vi "Save and Load Fixed-Point Settings.vi"() -> ()   [LabVIEW 2019]
doc: "This example demonstrates how to simulate the performance of a fixed-point LMS adaptive filter, obtain appropriate fixed-point settings from the simulation, save these settings to an XML file, and then load that XML file into LabVIEW.\n\nComplete the following steps to use this example.\n\n1. Select <b>Save to File</b> from the <b>Operation</b> pull-down menu and run this VI.\n\n2. In the dialog box that appears, specify a file name and click the <b>OK</b> button to save the fixed-point settings.\n\n3. Close and reopen this example.\n\n4. Select <b>Load from File</b> from the <b>Operation</b> pull-down menu and run this VI.\n \n5. In the dialog box that appears, navigate to the XML file you saved in Step 2 and click the <b>Open</b> button. This example then loads the fixed-point settings and displays the settings in <b>Fixed-Point Settings</b>."
uses:
  <vilib>/addons/Adaptive Filters/Utilities/AFT Fixed-Point Settings.ctl
  <vilib>/addons/Adaptive Filters/Utilities/AFT Algorithm.ctl
  <vilib>/addons/Adaptive Filters/Fixed-Point Simulation/LMS/AFT Simulate Fixed-Point FIR LMS.xnode
  <vilib>/addons/Adaptive Filters/NI_AdaptiveFilter.lvlib
  <vilib>/addons/Adaptive Filters/Utilities/AFT Simulation Info.ctl
panel:
  in  "Operation":enum16{"Save to File", "Load from File"}(ring)
  out "Coefficients":dbl[][](graph)
  out "Fixed-Point Settings":T1 {"algorithm" items=["LMS"]}
  out "Error Signal":dbl[](graph)
  # "Select Help>>Show Context Help and move the cursor over the VI icon of this example for more information."
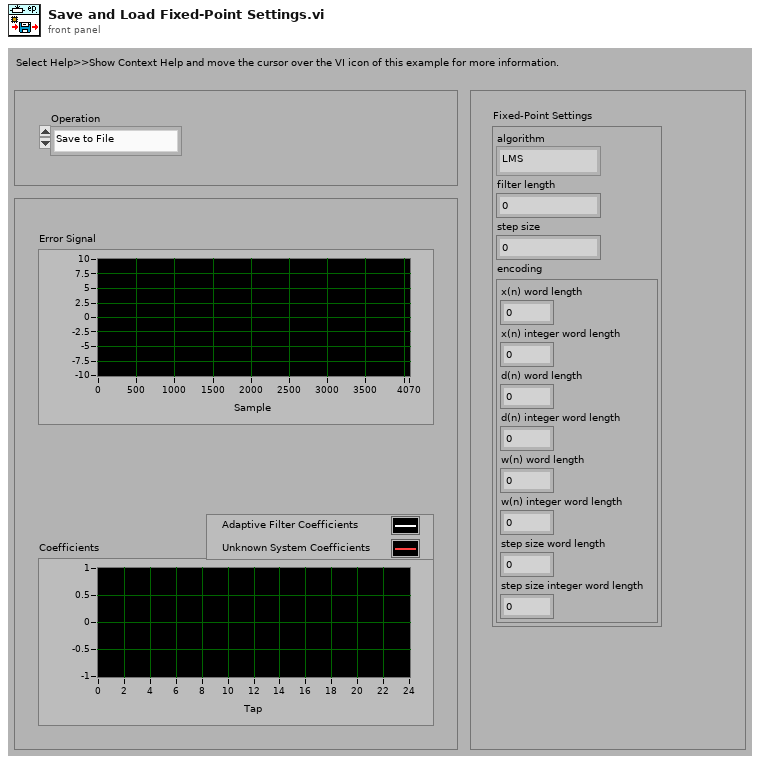
[diagram p1: front panel]
types:
  T1 = cluster{"algorithm":u16, "filter length":i32, "step size":dbl, "encoding":cluster{"x(n) word length":i32, "x(n) integer word length":i32, "d(n) word length":i32, "d(n) integer word length":i32, "w(n) word length":i32, "w(n) integer word length":i32, "step size word length":i32, "step size integer word length":i32}}
  T2 = typedef "NI_AdaptiveFilter.lvlib/AFT Fixed-Point Settings.ctl" = cluster{"algorithm":u16, "filter length":i32, "step size":dbl, "encoding":cluster{"x(n) word length":i32, "x(n) integer word length":i32, "d(n) word length":i32, "d(n) integer word length":i32, "w(n) word length":i32, "w(n) integer word length":i32, "step size word length":i32, "step size integer word length":i32}}
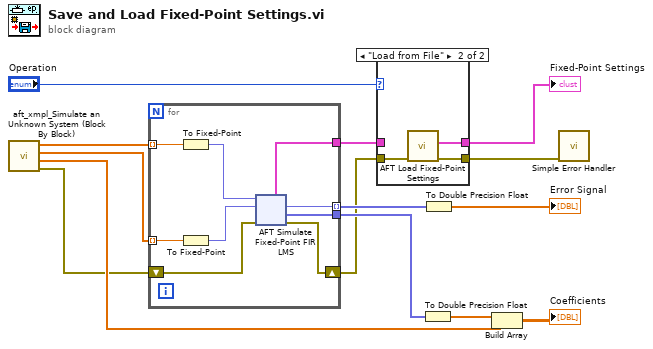
[diagram p0: block diagram]
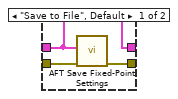
[diagram p2: hidden frame]
diagram:
  n1 = call "aft_xmpl_Simulate an Unknown System (Block By Block).vi"() -> ("error out"=w4:errorcluster, "unknown system coefficients"=w5:dbl[], "response signal"=w6:dbl[], "stimulus signal"=w7:dbl[])  [unwired: 4 in, 4 out]
  n2 = for {
    tunnel: w7 -> [w20] mode=indexing
    tunnel: w6 -> [w21] mode=indexing
    tunnel: [w23] -> w14 mode=indexing
    tunnel: [w22] -> w12
    tunnel: [w17] -> w11
    shift-right: [w16] -> w8
    shift-left: w4 -> [w15]
    n3 = To Fixed-Point(number=w20) -> (fixed-point=w19:fxp<+/-,24,4>)  [unwired: 1 out]
    n4 = To Fixed-Point(number=w21) -> (fixed-point=w18:fxp<+/-,24,4>)  [unwired: 1 out]
    n5 = xnode "AFT Simulate Fixed-Point FIR LMS"("x(n)"=w19, "d(n)"=w18, "error in (no error)"=w15) -> ("e(n)"=w23:fxp<+/-,24,4>, "coefficients"=w22:fxp<+/-,24,1>[], "fixed-point settings"=w17:T2, "error out"=w16:errorcluster)  [unwired: 2 in, 2 out]
  }
  n6 = case shown="\"Load from File\"" "Operation" {
    tunnel: w11 -> [w137 _]
    tunnel: [w139 w141] -> w1
    tunnel: w8 -> [w138 w142]
    tunnel: [w137 w140] -> w2
    frame "Save to File", Default {
      n7 = call <vilib>:"AFT Save Fixed-Point Settings.vi"("error in (no error)"=w138, "fixed-point settings"=w137) -> ("error out"=w139:errorcluster)  [unwired: 1 in, 8 out]
    }
    frame "Load from File" {
      n8 = call <vilib>:"AFT Load Fixed-Point Settings.vi"("error in (no error)"=w142) -> ("error out"=w141:errorcluster, "fixed-point settings"=w140:T2)  [unwired: 1 in, 8 out]
    }
  }
  "Fixed-Point Settings" <- w2
  n9 = To Double Precision Float(number=w12) -> (double precision float=w10:dbl[])
  n10 = To Double Precision Float(number=w14) -> (double precision float=→"Error Signal":dbl[])
  n11 = Build Array(w10, w5) -> (→"Coefficients":dbl[][])
  n12 = call <vilib>:"Simple Error Handler.vi"("error in (no error)"=w1) -> ()  [unwired: 4 in, 5 out]
